vi "Condition Map.vi"(6 "Name Refs.Name VI":refnum<vi>, 8 "error in":errorcluster, 9 "Conn Pane Terminals.Msg Output Indicator":i32[](array[numeric]), 10 "Conn Pane Terminals.Msg Control":i32[](array[numeric])) -> (0 "error out":errorcluster, 1 "Msg Output Terminal Map":T1, 2 "Msg Terminal Map":T3)   [LabVIEW 2025, in "_Msg Rescript.lvlib" / "_Msg Rescript.lvclass"]
uses:
  _Msg Rescript.lvclass
  _Msg Rescript.lvclass/_Msg Rescript.ctl
  Msg Terminal Attributes.ctl
  Msg Terminal Map.ctl
  Msg Output Terminal Attributes.ctl
  Msg Output Terminal Map.ctl
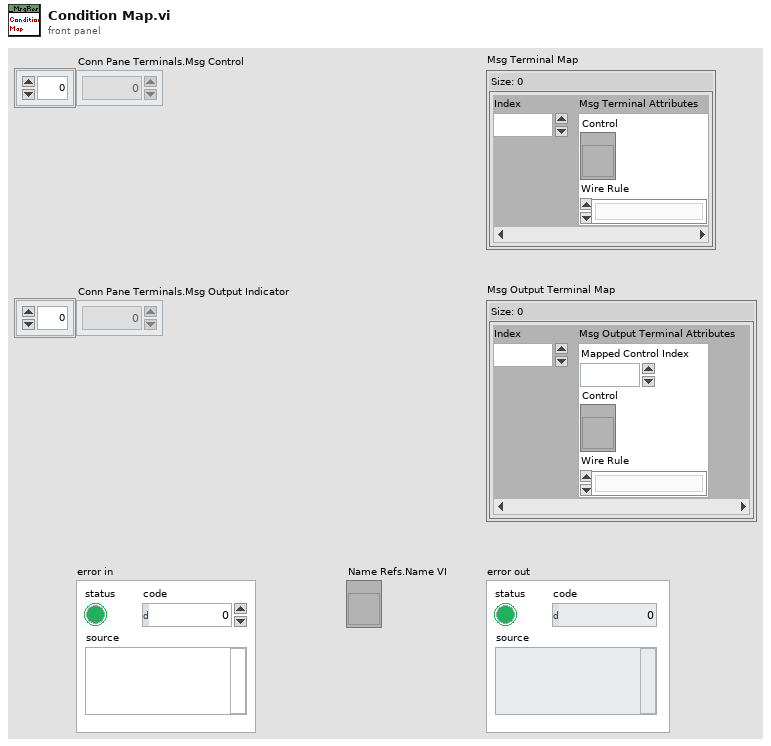
[diagram p1: front panel]
types:
  T1 = typedef "_Msg Rescript.lvlib/_Msg Rescript.lvclass/Msg Output Terminal Map.ctl" = map{i32, T2}
  T2 = typedef "_Msg Rescript.lvlib/_Msg Rescript.lvclass/Msg Output Terminal Attributes.ctl" = cluster{"Mapped Control Index":i32, "Control":refnum<vi>, "Wire Rule":enum16{"Invalid Wire Rule", "Required", "Recommended", "Optional", "Dynamic Dispatch"}}
  T3 = typedef "_Msg Rescript.lvlib/_Msg Rescript.lvclass/Msg Terminal Map.ctl" = map{i32, T4}
  T4 = typedef "_Msg Rescript.lvlib/_Msg Rescript.lvclass/Msg Terminal Attributes.ctl" = cluster{"Control":refnum<vi>, "Wire Rule":enum16{"Invalid Wire Rule", "Required", "Recommended", "Optional", "Dynamic Dispatch"}}
  T5 = enum16{"Invalid Wire Rule", "Required", "Recommended", "Optional", "Dynamic Dispatch"}[]
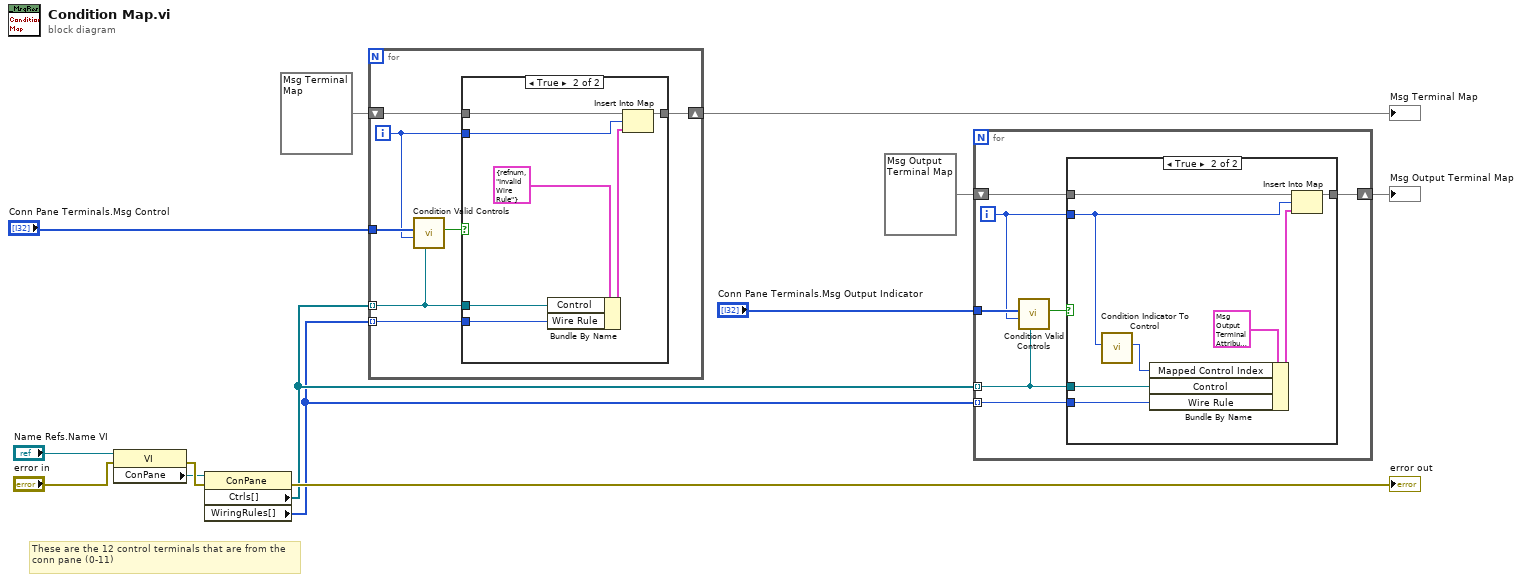
[diagram p0: block diagram]
diagram:
  # "These are the 12 control terminals that are from the conn pane (0-11)"
  n1 = property class="VI"(reference="Name Refs.Name VI", error in="error in") -> (error out=w12:errorcluster, "ConPane"=w11:refnum<vi>)  [unwired: 1 out]
  n2 = property class="ConPane"(reference=w11, error in=w12) -> (error out=→"error out":errorcluster, "Ctrls[]"=w3:refnum<vi>[], "WiringRules[]"=w2:T5)  [unwired: 1 out]
  n3 = for {
    tunnel: "Conn Pane Terminals.Msg Control" -> [w16]
    shift-right: [w20] -> w7
    shift-left: T3 {} ("Msg Terminal Map") -> [w19]
    tunnel: w3 -> [w14] mode=indexing
    tunnel: w2 -> [w18] mode=indexing
    i -> [w15]
    n4 = call "Condition Valid Controls.vi"("Ctl Refnum"=w14, "Terminal Index"=w15, "Control Terminals"=w16) -> ("Valid"=w17:bool)  [unwired: 8 in]
    n5 = case shown="True" w17 {
      tunnel: [w21 w28] -> w20
      tunnel: w19 -> [w21 w27]
      tunnel: w18 -> [_ w26]
      tunnel: w15 -> [_ w25]
      tunnel: w14 -> [_ w24]
      frame False {
      }
      frame True {
        n6 = Bundle By Name(cluster=T4 {"Control"=refnum, "Wire Rule"=enum."Invalid Wire Rule"} ("value"), "Control"=w24, "Wire Rule"=w26) -> (w22:T4)
        n7 = Insert Into Map(map in=w27, key=w25, value=w22) -> (map out=w28:T3)  [unwired: 2 out]
      }
    }
  }
  "Msg Terminal Map" <- w7
  n8 = for {
    tunnel: "Conn Pane Terminals.Msg Output Indicator" -> [w31]
    shift-right: [w35] -> w4
    shift-left: T1 {} ("Msg Output Terminal Map") -> [w34]
    tunnel: w3 -> [w29] mode=indexing
    tunnel: w2 -> [w33] mode=indexing
    i -> [w30]
    n9 = call "Condition Valid Controls.vi"("Ctl Refnum"=w29, "Terminal Index"=w30, "Control Terminals"=w31) -> ("Valid"=w32:bool)  [unwired: 8 in]
    n10 = case shown="True" w32 {
      tunnel: [w36 w44] -> w35
      tunnel: w34 -> [w36 w43]
      tunnel: w33 -> [_ w42]
      tunnel: w30 -> [_ w38]
      tunnel: w29 -> [_ w41]
      frame False {
      }
      frame True {
        n11 = call "Condition Indicator To Control.vi"("Index"=w38) -> ("Mapped Control Index"=w37:i32)  [unwired: 10 in]
        n12 = Bundle By Name(cluster=T2 {"Mapped Control Index"=0, "Control"=refnum, "Wire Rule"=enum."Invalid Wire Rule"} ("value"), "Mapped Control Index"=w37, "Control"=w41, "Wire Rule"=w42) -> (w39:T2)
        n13 = Insert Into Map(map in=w43, key=w38, value=w39) -> (map out=w44:T1)  [unwired: 2 out]
      }
    }
  }
  "Msg Output Terminal Map" <- w4
